vi "Test init from Config file.vi"() -> ()   [LabVIEW 2009, in "POLARIS BME DG.lvlib"]
uses:
  POLARIS BME DG.lvlib
  LV-BME Interface/ChnlSettings.ctl
  DG Classes/BME_DG_System/BME_DG_System.lvclass
  DG Classes/BME_DG_Base/BME_DG_Base.lvclass
  DG Classes/BME_DG_Chnl/BME_DG_Chnl.lvclass
panel:
  out "Created new":bool
  in  "pathCalFiles":path
  in  "pathParameterFile":path
  out "stop error":errorcluster
  out "Problem Chnls out":string[](array[string])
  out "DelayFormulas":string[](array[string])=[" 10000.0095", "Delay Offset +0.819", "Pulspicker On + 0.013"]
  in  "Reset Error":bool
  out "error out":errorcluster
  in  "Update Delay formula":bool=TRUE
  in  "DelayFormula":string=" 10000.0095"
  in  "Aknowledge interrupts":bool=TRUE
  in  "stop 3":bool=TRUE
  in  "SetDelay":bool=TRUE
  in  "UpdateChnl":bool=TRUE
  in  "ChnlParameter":T2 {"ChnParam2write"."Delay (µs)" min=0.0 max=100000000.0 format="%.5f"}
  out "CountsRemains":i32=2147483647
  out "TriggerCounters":i32[](array[numeric])=[281, 0, 0, 0, -533591008, 0, 0, 0, 0]
  out "Interrupts":u32[](array[numeric])=[11153, 10240, 10240, 10240, 11008, 11008, 10240, 10240, 10240] format="%b"
  out "RemainingTriggers":T3(array[cluster])=[[{"Time Stamp"=timestamp(3421911180.6875 s since 1904-01-01), "Numeric"=1}, {"Time Stamp"=timestamp(3421911180.6875 s since 1904-01-01), "Numeric"=1}, {"Time Stamp"=timestamp(3421911180.6875 s since 1904-01-01), "Numeric"=1}, {"Time Stamp"=timestamp(3421911180.6875 s since 1904-01-01), "Numeric"=1}, {"Time Stamp"=timestamp(3421911180.6875 s since 1904-01-01), "Numeric"=9}, {"Time Stamp"=timestamp(3421911180.6875 s since 1904-01-01), "Numeric"=1}, {"Time Stamp"=timestamp(3421911180.6875 s since 1904-01-01), "Numeric"=1}, {"Time Stamp"=timestamp(3421911180.6875 s since 1904-01-01), "Numeric"=1}, {"Time Stamp"=timestamp(3421911180.6875 s since 1904-01-01), "Numeric"=1}], [{"Time Stamp"=timestamp(3421911180.6875 s since 1904-01-01), "Numeric"=10}, {"Time Stamp"=timestamp(3421911180.6875 s since 1904-01-01), "Numeric"=1}, {"Time Stamp"=timestamp(3421911180.6875 s since 1904-01-01), "Numeric"=1}, {"Time Stamp"=timestamp(3421911180.6875 s since 1904-01-01), "Numeric"=1}, {"Time Stamp"=timestamp(3421911180.6875 s since 1904-01-01), "Numeric"=9}, {"Time Stamp"=timestamp(3421911180.6875 s since 1904-01-01), "Numeric"=1}, {"Time Stamp"=timestamp(3421911180.6875 s since 1904-01-01), "Numeric"=1}, {"Time Stamp"=timestamp(3421911180.6875 s since 1904-01-01), "Numeric"=1}, {"Time Stamp"=timestamp(3421911180.6875 s since 1904-01-01), "Numeric"=1}], [{"Time Stamp"=timestamp(3421911180.6875 s since 1904-01-01), "Numeric"=10}, {"Time Stamp"=timestamp(3421911180.6875 s since 1904-01-01), "Numeric"=1}, {"Time Stamp"=timestamp(3421911180.6875 s since 1904-01-01), "Numeric"=1}, {"Time Stamp"=timestamp(3421911180.6875 s since 1904-01-01), "Numeric"=1}, {"Time Stamp"=timestamp(3421911180.6875 s since 1904-01-01), "Numeric"=609}, {"Time Stamp"=timestamp(3421911180.6875 s since 1904-01-01), "Numeric"=1}, {"Time Stamp"=timestamp(3421911180.6875 s since 1904-01-01), "Numeric"=1}, {"Time Stamp"=timestamp(3421911180.6875 s since 1904-01-01), "Numeric"=1}, {"Time Stamp"=timestamp(3421911180.6875 s since 1904-01-01), "Numeric"=1}]] {"Time Stamp" format="%<%I:%M:%S%3u %p>T"}
  in  "stop 2":bool=TRUE
  in  "ReadStatus":bool=TRUE
  in  "Activate":bool=TRUE
  in  "ResetModuloCounters":bool=TRUE
  in  "TriggerModulo":u32=4
  out "Modulo Settings":u32[](array[numeric])=[1, 10, 10]
  out "Chnls":T1[](array[typedef])=[{" Delay (µs)"=10000.0095, "On?"=TRUE, "PositiveVoltage?"=TRUE, "50OhmTerminated? "=TRUE, "25OhmOutput?"=FALSE}, {" Delay (µs)"=10000.829, "On?"=TRUE, "PositiveVoltage?"=TRUE, "50OhmTerminated? "=TRUE, "25OhmOutput?"=FALSE}, {" Delay (µs)"=10000.843, "On?"=TRUE, "PositiveVoltage?"=TRUE, "50OhmTerminated? "=TRUE, "25OhmOutput?"=FALSE}] {"Delay (µs)" min=0.0 max=100000000.0 format="%.5f"}
  in  "Selected Chnl":u16(ring) items=["MA", "MB", "MC", "MD", "ME", "MF"]
  in  "Selected Card":u16(ring) items=["Master", "Slave"]
  in  "STOP":bool
  in  "ChnParam2write":T1={" Delay (µs)"=0.0, "On?"=TRUE, "PositiveVoltage?"=TRUE, "50OhmTerminated? "=TRUE, "25OhmOutput?"=FALSE} {"Delay (µs)" min=0.0 max=100000000.0 format="%.5f"}
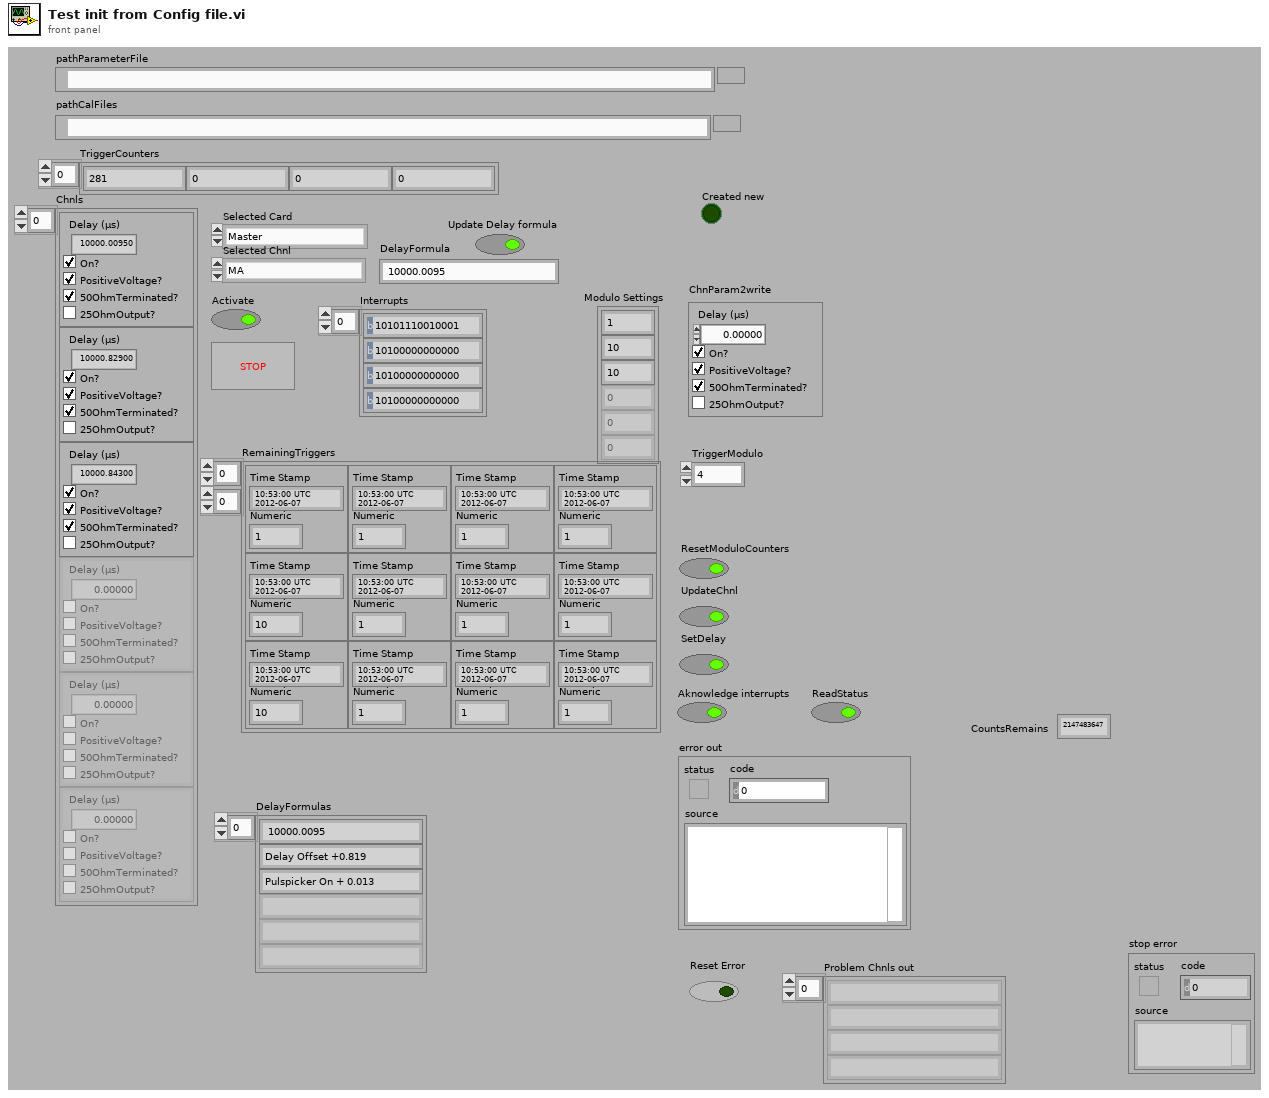
[diagram p1: front panel]
types:
  T1 = typedef "POLARIS BME DG.lvlib/ChnlSettings.ctl" = cluster{" Delay (µs)":dbl, "On?":bool, "PositiveVoltage?":bool, "50OhmTerminated? ":bool, "25OhmOutput?":bool}
  T2 = cluster{"ChnlName":string, "ChnParam2write":T1, "TriggerModulo":u32}
  T3 = cluster{"Time Stamp":timestamp, "Numeric":i32}[][]
  T4 = typedef "POLARIS BME DG.lvlib/BME_DG_MasterOrSlave.ctl" = enum16{"Unknown", "Master", "Slave"}
  T5 = enum8{"Enabled", "Disabled", "Disabled and Grayed Out"}
  T6 = typedef "POLARIS BME DG.lvlib/BME_DG_TriggerSettings.ctl" = cluster{"Clock Source":T7, " clock devide by":u32, "TriggerEnabled?":bool, "Trigger devide by":i32, "InputTerminated?":bool, "Inhibit(µs)":dbl, "TriggerLevel":dbl, "PresetValue":i32, "InternalTrigger?":bool, "InternalArm?":bool, "SWTrigger?":bool, "RisingEdge?":bool, "StopOnPreset?":bool, "ResetWhenDone?":bool, "Gate Divider":i32, "PositiveGate?":bool}
  T7 = typedef "POLARIS BME DG.lvlib/ClockSource.ctl" = i32
  T8 = cluster{"ChnlName":string, "ChnParam2write":T1, "TriggerModulo":u32}[]
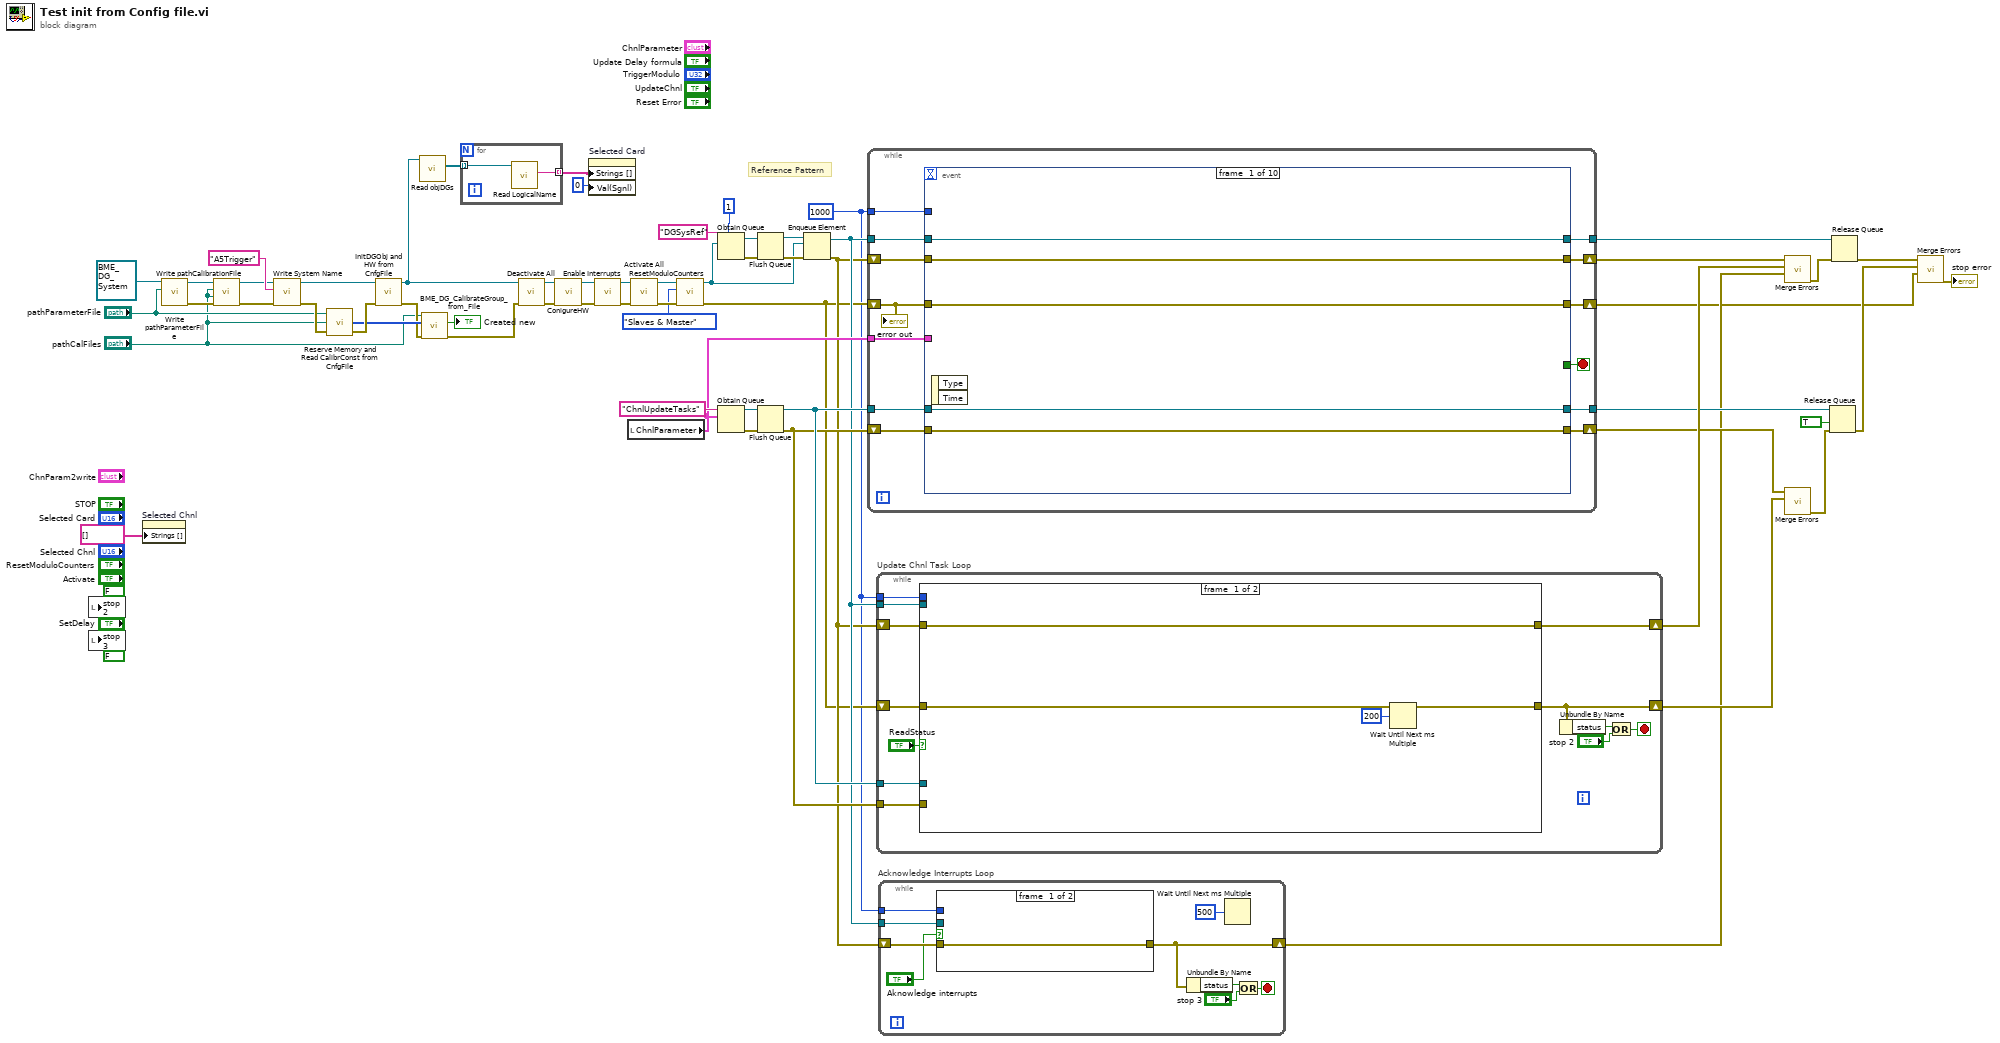
[diagram p0: block diagram]
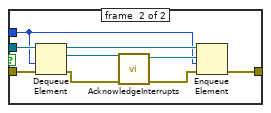
[diagram p2: hidden frame]
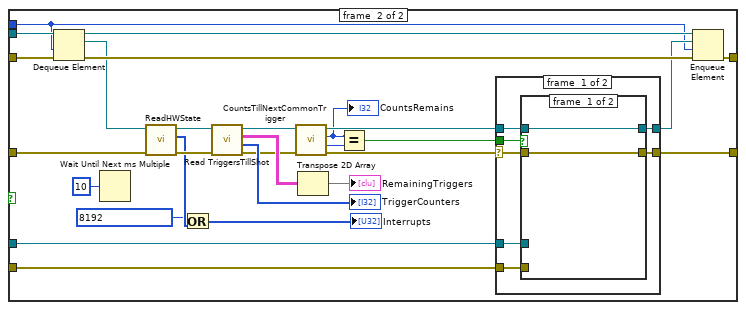
[diagram p3: hidden frame]
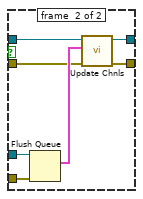
[diagram p4: hidden frame]
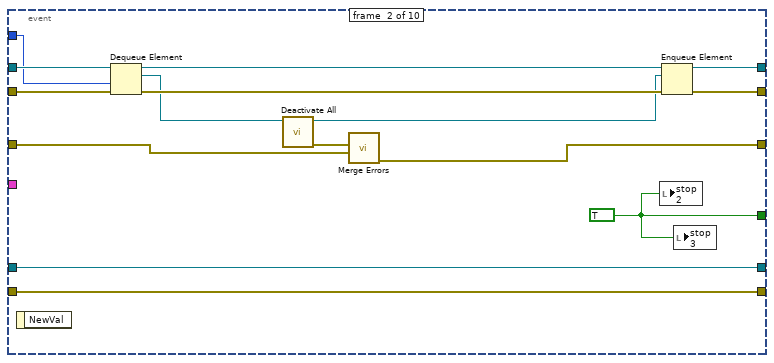
[diagram p6: hidden frame]
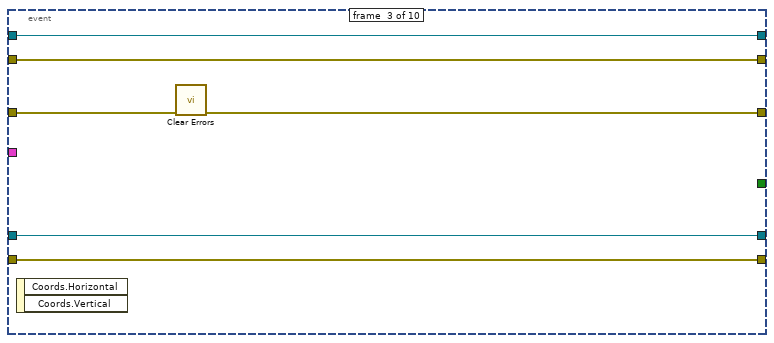
[diagram p7: hidden frame]
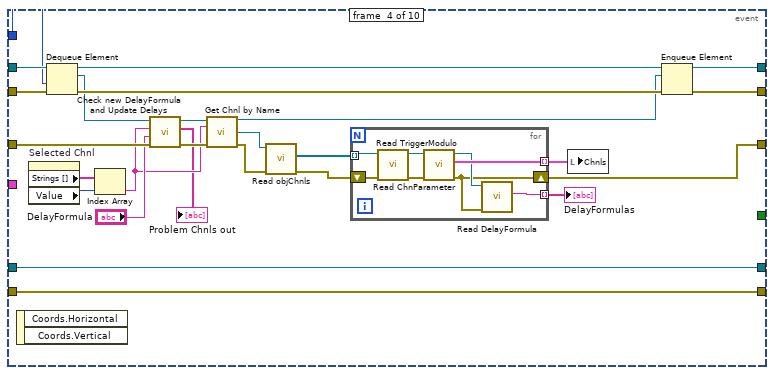
[diagram p8: hidden frame]
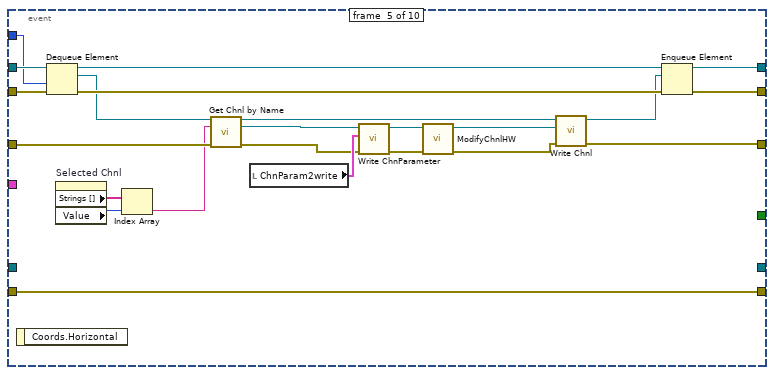
[diagram p9: hidden frame]
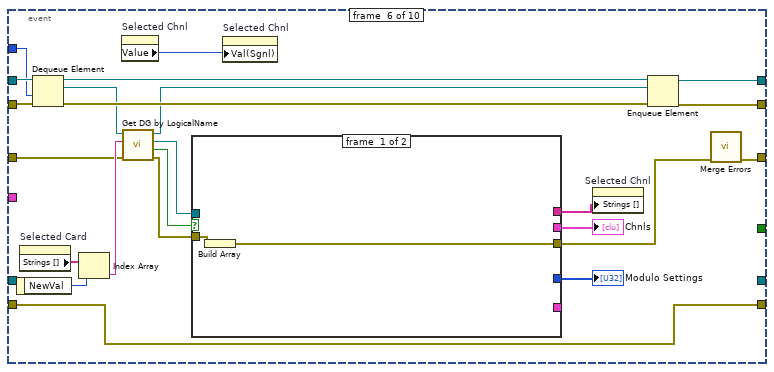
[diagram p10: hidden frame]
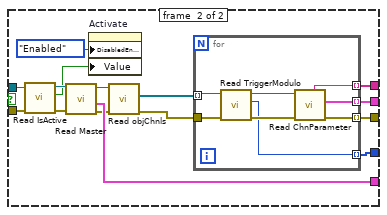
[diagram p11: hidden frame]
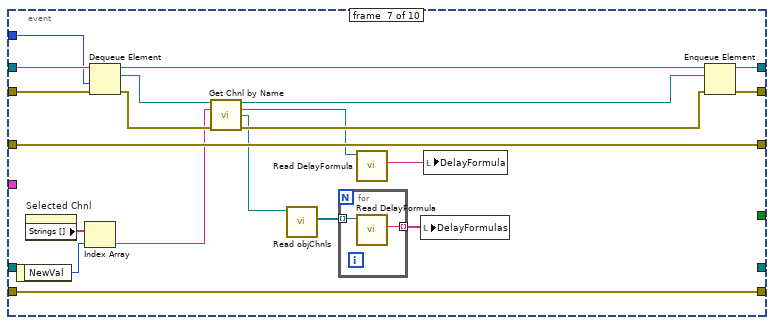
[diagram p12: hidden frame]
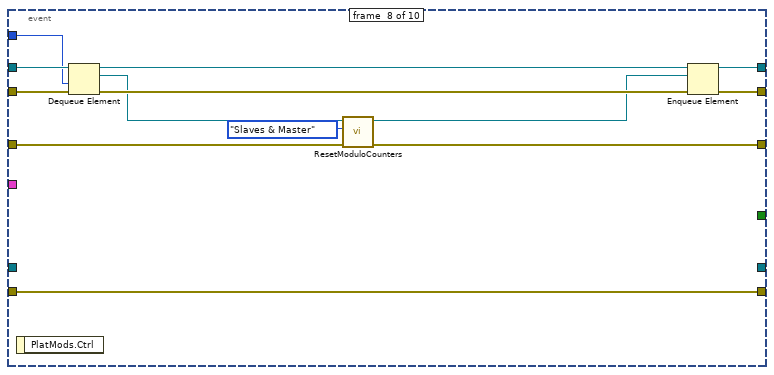
[diagram p13: hidden frame]
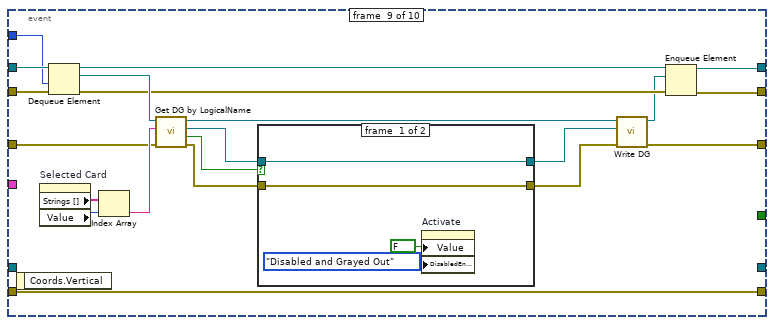
[diagram p14: hidden frame]
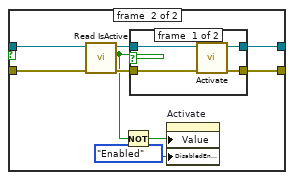
[diagram p15: hidden frame]
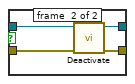
[diagram p16: hidden frame]
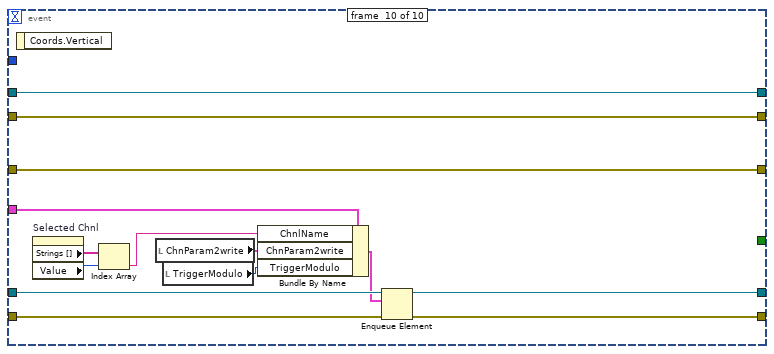
[diagram p17: hidden frame]
diagram:
  w17 = 1000 ("timeout in ms (-1)")
  # "Reference Pattern"
  n1 = local write "stop 2"(FALSE ("stop 2")) -> ()
  n2 = local write "stop 3"(FALSE ("stop 3")) -> ()
  n3 = property on="Selected Chnl" class="Ring (strict)"("Strings []"=string[] []) -> ()  [unwired: 2 in, 2 out]
  n4 = call-dynamic "Write pathParameterFile.vi"("pathParameterFile"="pathParameterFile", "BME_DG_System in"=refnum<class "BME_DG_System.lvclass"> refnum ("BME_DG_System.lvclass")) -> ("error out"=w13:errorcluster, "BME_DG_System out"=w15:refnum<class "BME_DG_System.lvclass">)  [unwired: 8 in]
  n5 = call-dynamic "Write pathCalibrationFile.vi"("error in (no error)"=w13, "pathModulesCal"="pathCalFiles", "pathBMEG0xCal"="pathCalFiles", "BME_DG_System in"=w15) -> ("error out"=w12:errorcluster, "BME_DG_System out"=w14:refnum<class "BME_DG_System.lvclass">)  [unwired: 6 in]
  n6 = call "Write System Name.vi"("error in (no error)"=w12, "log Name"="A5Trigger", "BME_DG_System in"=w14) -> ("error out"=w11:errorcluster, "BME_DG_System out"=w18:refnum<class "BME_DG_System.lvclass">)  [unwired: 7 in]
  n7 = call "Reserve Memory and Read CalibrConst from CnfgFile.vi"("error out 2"=w11, "pathCalibrConsts"="pathCalFiles", "pathConfigFile"="pathParameterFile") -> ("error out"=w10:errorcluster, "Master or Slave?"=w7:T4[])  [unwired: 1 in]
  n8 = call "InitDGObj and HW from CnfgFile.vi"("error in"=w10, "BME_DG_System in"=w18) -> ("error IO"=w6:errorcluster, "BME_DG_System Out"=w3:refnum<class "BME_DG_System.lvclass">)  [unwired: 4 in]
  n9 = call "Read objDGs.vi"("BME_DG_System in"=w3) -> ("objDGs"=w2:refnum<class "BME_DG_Base.lvclass">[])  [unwired: 8 in, 2 out]
  n10 = call "BME_DG_CalibrateGroup_from_File.vi"("error in (no error)"=w6, "p_MasterOrSlave"=w7, "Path"="pathCalFiles") -> ("error out"=w4:errorcluster, "Created new"=→"Created new":bool)  [unwired: 7 in]
  n11 = for {
    tunnel: w2 -> [w64] mode=indexing
    tunnel: [w63] -> w1 mode=indexing
    n12 = call "Read LogicalName.vi"("BME_DG_Base in"=w64) -> ("LogicalName"=w63:string)  [unwired: 8 in, 2 out]
  }
  n13 = call "Deactivate All.vi"("error in (no error)"=w4, "BME_DG_System in"=w3) -> ("error out"=w37:errorcluster, "BME_DG_System out"=w38:refnum<class "BME_DG_System.lvclass">)  [unwired: 8 in]
  n14 = call "ConigureHW.vi"("error in (no error)"=w37, "BME_DG_System in"=w38) -> ("error out"=w35:errorcluster, "BME_DG_System out"=w36:refnum<class "BME_DG_System.lvclass">)  [unwired: 8 in]
  n15 = property on="Selected Card" class="Ring (strict)"("Strings []"=w1, "Val(Sgnl)"=u16 0 ("Value (Signaling)")) -> ()  [unwired: 2 in, 2 out]
  n16 = call "Enable Interrupts.vi"("error in (no error)"=w35, "BME_DG_System in"=w36) -> ("error out"=w29:errorcluster, "BME_DG_System out"=w30:refnum<class "BME_DG_System.lvclass">)  [unwired: 8 in]
  n17 = local read "ChnlParameter"() -> (w46:T2)
  n18 = call "Activate All.vi"("error in (no error)"=w29, "BME_DG_System in"=w30) -> ("error out"=w26:errorcluster, "BME_DG_System out"=w28:refnum<class "BME_DG_System.lvclass">)  [unwired: 8 in]
  n19 = call "ResetModuloCounters.vi"("error in (no error)"=w26, "Enum"=enum16{"Slaves only", "Slaves & Master"}."Slaves & Master", "BME_DG_System in"=w28) -> ("error out"=w25:errorcluster, "BME_DG_System out"=w27:refnum<class "BME_DG_System.lvclass">)  [unwired: 7 in]
  n20 = Obtain Queue(max queue size (-1, unlimited)=1, name (unnamed)="DGSysRef", element data type=w27) -> (queue out=w54:refnum<queue>, error out=w52:errorcluster)  [unwired: 2 in, 1 out]
  n21 = Obtain Queue(name (unnamed)="ChnlUpdateTasks", element data type=w46) -> (queue out=w47:refnum<queue>, error out=w48:errorcluster)  [unwired: 3 in, 1 out]
  n22 = Flush Queue(queue=w54, error in (no error)=w52) -> (queue out=w53:refnum<queue>, error out=w51:errorcluster)  [unwired: 1 out]
  n23 = Flush Queue(queue=w47, error in (no error)=w48) -> (queue out=w43:refnum<queue>, error out=w42:errorcluster)  [unwired: 1 out]
  n24 = Enqueue Element(queue=w53, element=w27, error in (no error)=w51) -> (queue out=w34:refnum<queue>, error out=w33:errorcluster)  [unwired: 1 in, 1 out]
  n25 = while {
    shift-right: [w73] -> w16
    shift-left: w25 -> [w75]
    shift-right: [w71] -> w57
    shift-left: w33 -> [w72]
    tunnel: w34 -> [w76]
    tunnel: [w74] -> w59
    tunnel: w43 -> [w70]
    tunnel: w46 -> [w69]
    tunnel: [w67] -> w45
    shift-right: [w66] -> w41
    shift-left: w42 -> [w68]
    tunnel: w17 -> [w65]
    stop <- w77 stop-if-true
    n26 = event shown="[5] \"Selected Card\": Value Change" {
      selector: _ -> [_ _ _ _ _ _ _ _ _ _]
      dyn-events: _ -> [_ _ _ _ _ _ _ _ _ _]
      timeout: _ -> [_ _ _ _ _ _ _ _ _ _]
      tunnel: [_ w86 _ _ _ _ _ _ _ _] -> w77
      tunnel: w76 -> [w82 w95 w102 w128 w159 w172 w223 w243 w253 w299]
      tunnel: w75 -> [w81 w84 w103 w120 w150 w180 w228 w233 w261 w298]
      tunnel: [w82 w91 w102 w124 w155 w170 w221 w238 w247 w299] -> w74
      tunnel: [w81 w85 w98 w108 w139 w165 w228 w234 w254 w298] -> w73
      tunnel: w72 -> [w80 w94 w101 w127 w158 w171 w222 w241 w252 w295]
      tunnel: [w80 w92 w101 w125 w156 w169 w220 w239 w246 w295] -> w71
      tunnel: w70 -> [w79 w88 w100 w123 _ _ _ _ _ w290]
      tunnel: w69 -> [_ _ _ _ _ _ _ _ _ w294]
      tunnel: w68 -> [w78 w87 w99 w122 w154 w163 w227 w237 w245 w288]
      tunnel: [w79 w88 w100 w123 _ _ _ _ _ w287] -> w67
      tunnel: [w78 w87 w99 w122 w154 w163 w227 w237 w245 w286] -> w66
      tunnel: w65 -> [_ w83 _ w104 w138 w161 w209 w231 w244 _]
      event #0 {
        n27 = event-data() -> ()  [unwired: 1 in, 2 out]
      }
      event #1 {
        w86 = TRUE
        n28 = event-data() -> ()  [unwired: 1 in, 1 out]
        n29 = Dequeue Element(queue=w95, timeout in ms (-1)=w83, error in (no error)=w94) -> (queue out=w96:refnum<queue>, element=w89:refnum<class "BME_DG_System.lvclass">, error out=w93:errorcluster)  [unwired: 1 out]
        n30 = call "Deactivate All.vi"("BME_DG_System in"=w89) -> ("error out"=w97:errorcluster, "BME_DG_System out"=w90:refnum<class "BME_DG_System.lvclass">)  [unwired: 9 in]
        n31 = call <vilib>:"Merge Errors.vi"("error in 3 (no error)"=w84, "error in 2 (no error)"=w97) -> ("error out"=w85:errorcluster)  [unwired: 5 in]
        n32 = local write "stop 2"(w86) -> ()
        n33 = Enqueue Element(queue=w96, element=w90, error in (no error)=w93) -> (queue out=w91:refnum<queue>, error out=w92:errorcluster)  [unwired: 1 in, 1 out]
        n34 = local write "stop 3"(w86) -> ()
      }
      event #2 {
        n35 = event-data() -> ()  [unwired: 1 in, 2 out]
        n36 = call <vilib>:"Clear Errors.vi"("error in (no error)"=w103) -> ("error out"=w98:errorcluster)  [unwired: 6 in]
      }
      event #3 {
        n37 = event-data() -> ()  [unwired: 1 in, 2 out]
        n38 = property on="Selected Chnl" class="Ring (strict)"() -> ("Strings []"=w118:string[], "Value"=w119:u16)  [unwired: 2 in, 2 out]
        n39 = Dequeue Element(queue=w128, timeout in ms (-1)=w104, error in (no error)=w127) -> (queue out=w129:refnum<queue>, element=w121:refnum<class "BME_DG_System.lvclass">, error out=w126:errorcluster)  [unwired: 1 out]
        n40 = Index Array(array=w118, index=w119) -> (element=w107:string)
        n41 = call "Check new DelayFormula and Update Delays.vi"("error in (no error)"=w120, "Delay Formula"="DelayFormula", "ChnlName"=w107, "BME_DG_System in"=w121) -> ("error out"=w110:errorcluster, "Problem Chnls out"=→"Problem Chnls out":string[], "BME_DG_System out"=w112:refnum<class "BME_DG_System.lvclass">)  [unwired: 5 in]
        n42 = call "Get Chnl by Name.vi"("BME_DG_System in"=w112, "Chnl Name"=w107, "error in (no error)"=w110) -> ("BME_DG_System out"=w111:refnum<class "BME_DG_System.lvclass">, "Owner DG"=w113:refnum<class "BME_DG_Base.lvclass">, "error out"=w109:errorcluster)  [unwired: 7 in, 3 out]
        n43 = call-dynamic "Read objChnls.vi"("error in (no error)"=w109, "BME_DG_Base in"=w113) -> ("error out"=w114:errorcluster, "objChnls"=w116:refnum<class "BME_DG_Chnl.lvclass">[])  [unwired: 6 in, 2 out]
        n44 = for {
          tunnel: w116 -> [w136] mode=indexing
          tunnel: [w137] -> w115 mode=indexing
          shift-right: [w131] -> w108
          shift-left: w114 -> [w134]
          tunnel: [w130] -> w106 mode=indexing
          n45 = call-dynamic "Read TriggerModulo.vi"("error in (no error)"=w134, "BME_DG_Chnl in"=w136) -> ("error out"=w133:errorcluster, "BME_DG_Chnl out"=w135:refnum<class "BME_DG_Chnl.lvclass">)  [unwired: 7 in, 1 out]
          n46 = call-dynamic "Read ChnParameter.vi"("error in (no error)"=w133, "BME_DG_Chnl in"=w135) -> ("error out"=w131:errorcluster, "ChnParemater"=w137:T1, "BME_DG_Chnl out"=w132:refnum<class "BME_DG_Chnl.lvclass">)  [unwired: 4 in, 3 out]
          n47 = call-dynamic "Read DelayFormula.vi"("error in (no error)"=w131, "BME_DG_Chnl in"=w132) -> ("DelayFormula"=w130:string)  [unwired: 7 in, 2 out]
        }
        "DelayFormulas" <- w106
        n48 = local write "Chnls"(w115) -> ()
        n49 = Enqueue Element(queue=w129, element=w111, error in (no error)=w126) -> (queue out=w124:refnum<queue>, error out=w125:errorcluster)  [unwired: 1 in, 1 out]
      }
      event #4 {
        n50 = event-data() -> ()  [unwired: 1 in, 1 out]
        n51 = Dequeue Element(queue=w159, timeout in ms (-1)=w138, error in (no error)=w158) -> (queue out=w160:refnum<queue>, element=w151:refnum<class "BME_DG_System.lvclass">, error out=w157:errorcluster)  [unwired: 1 out]
        n52 = property on="Selected Chnl" class="Ring (strict)"() -> ("Strings []"=w152:string[], "Value"=w153:u16)  [unwired: 2 in, 2 out]
        n53 = Index Array(array=w152, index=w153) -> (element=w149:string)
        n54 = call "Get Chnl by Name.vi"("BME_DG_System in"=w151, "Chnl Name"=w149, "error in (no error)"=w150) -> ("BME_DG_System out"=w145:refnum<class "BME_DG_System.lvclass">, "BME_DG_Chnl"=w148:refnum<class "BME_DG_Chnl.lvclass">, "error out"=w146:errorcluster)  [unwired: 7 in, 3 out]
        n55 = local read "ChnParam2write"() -> (w147:T1)
        n56 = call-dynamic "Write ChnParameter.vi"("error in (no error)"=w146, "ChnParemater"=w147, "BME_DG_Chnl in"=w148) -> ("error out"=w142:errorcluster, "BME_DG_Chnl out"=w143:refnum<class "BME_DG_Chnl.lvclass">)  [unwired: 7 in]
        n57 = call-dynamic "ModifyChnlHW.vi"("error in (no error)"=w142, "BME_DG_Chnl in"=w143) -> ("error out"=w140:errorcluster, "BME_DG_Chnl out"=w141:refnum<class "BME_DG_Chnl.lvclass">)  [unwired: 8 in]
        n58 = call "Write Chnl.vi"("error in (no error)"=w140, "BME_DG_Chnl.lvclass"=w141, "BME_DG_System in"=w145) -> ("error out"=w139:errorcluster, "BME_DG_System out"=w144:refnum<class "BME_DG_System.lvclass">)  [unwired: 7 in]
        n59 = Enqueue Element(queue=w160, element=w144, error in (no error)=w157) -> (queue out=w155:refnum<queue>, error out=w156:errorcluster)  [unwired: 1 in, 1 out]
      }
      event #5 {
        n60 = event-data() -> ("NewVal"=w182:u16)  [unwired: 1 in]
        n61 = property on="Selected Card" class="Ring (strict)"() -> ("Strings []"=w183:string[])  [unwired: 2 in, 2 out]
        n62 = Dequeue Element(queue=w172, timeout in ms (-1)=w161, error in (no error)=w171) -> (queue out=w173:refnum<queue>, element=w168:refnum<class "BME_DG_System.lvclass">, error out=w174:errorcluster)  [unwired: 1 out]
        n63 = Index Array(array=w183, index=w182) -> (element=w181:string)
        n64 = property on="Selected Chnl" class="Ring (strict)"() -> ("Value"=w162:u16)  [unwired: 2 in, 2 out]
        n65 = call "Get DG by LogicalName.vi"("error in (no error)"=w180, "LogicalName"=w181, "BME_DG_System in"=w168) -> ("error out"=w166:errorcluster, "found?"=w179:bool, "BME_DG_Base.lvclass"=w178:refnum<class "BME_DG_Base.lvclass">, "BME_DG_System out"=w167:refnum<class "BME_DG_System.lvclass">)  [unwired: 5 in]
        n66 = case shown="True" w179 {
          tunnel: w178 -> [_ w193]
          tunnel: [_ w200] -> w177
          tunnel: [_ w199] -> w176
          tunnel: [_ w198] -> _
          tunnel: [_ w194] -> w175
          tunnel: w166 -> [w185 w190]
          tunnel: [w184 w188] -> w164
          frame #0 {
            n67 = Build Array(w185) -> (w184:errorcluster[])
          }
          frame #1 {
            n68 = call-dynamic "Read IsActive.vi"("error in (no error)"=w190, "BME_DG_Base in"=w193) -> ("error out"=w191:errorcluster, "Active?"=w186:bool, "BME_DG_Base out"=w192:refnum<class "BME_DG_Base.lvclass">)  [unwired: 7 in]
            n69 = call-dynamic "Read Master.vi"("error in (no error)"=w191, "BME_DG_Base in"=w192) -> ("error out"=w195:errorcluster, "TriggerSettings"=w198:T6, "BME_DG_Base out"=w196:refnum<class "BME_DG_Base.lvclass">)  [unwired: 6 in, 1 out]
            n70 = property on="Activate" class="Bool (strict)"("DisabledEnum"=T5."Enabled" ("Disabled"), "Value"=w186) -> ()  [unwired: 2 in, 2 out]
            n71 = call-dynamic "Read objChnls.vi"("error in (no error)"=w195, "BME_DG_Base in"=w196) -> ("error out"=w189:errorcluster, "objChnls"=w197:refnum<class "BME_DG_Chnl.lvclass">[])  [unwired: 6 in, 2 out]
            n72 = for {
              tunnel: w197 -> [w206] mode=indexing
              tunnel: [w208] -> w200 mode=indexing
              tunnel: [w207] -> w199 mode=indexing
              tunnel: [w201] -> w194 mode=indexing
              tunnel: w189 -> [w204]
              tunnel: [w202] -> w188 mode=indexing
              n73 = call-dynamic "Read TriggerModulo.vi"("error in (no error)"=w204, "BME_DG_Chnl in"=w206) -> ("error out"=w203:errorcluster, "TriggerModulo"=w201:i32, "BME_DG_Chnl out"=w205:refnum<class "BME_DG_Chnl.lvclass">)  [unwired: 7 in]
              n74 = call-dynamic "Read ChnParameter.vi"("error in (no error)"=w203, "BME_DG_Chnl in"=w205) -> ("error out"=w202:errorcluster, "ChnParemater"=w207:T1, "Name"=w208:string)  [unwired: 4 in, 3 out]
            }
          }
        }
        "Chnls" <- w176
        "Modulo Settings" <- w175
        n75 = property on="Selected Chnl" class="Ring (strict)"("Val(Sgnl)"=w162) -> ()  [unwired: 2 in, 2 out]
        n76 = property on="Selected Chnl" class="Ring (strict)"("Strings []"=w177) -> ()  [unwired: 2 in, 2 out]
        n77 = Enqueue Element(queue=w173, element=w167, error in (no error)=w174) -> (queue out=w170:refnum<queue>, error out=w169:errorcluster)  [unwired: 1 in, 1 out]
        n78 = call <vilib>:"Merge Errors.vi"("error array in"=w164) -> ("error out"=w165:errorcluster)  [unwired: 6 in]
      }
      event #6 {
        n79 = event-data() -> ("NewVal"=w225:u16)  [unwired: 1 in]
        n80 = property on="Selected Chnl" class="Ring (strict)"() -> ("Strings []"=w226:string[])  [unwired: 2 in, 2 out]
        n81 = Index Array(array=w226, index=w225) -> (element=w215:string)
        n82 = Dequeue Element(queue=w223, timeout in ms (-1)=w209, error in (no error)=w222) -> (queue out=w224:refnum<queue>, element=w216:refnum<class "BME_DG_System.lvclass">, error out=w218:errorcluster)  [unwired: 1 out]
        n83 = call "Get Chnl by Name.vi"("BME_DG_System in"=w216, "Chnl Name"=w215, "error in (no error)"=w218) -> ("BME_DG_System out"=w219:refnum<class "BME_DG_System.lvclass">, "BME_DG_Chnl"=w213:refnum<class "BME_DG_Chnl.lvclass">, "Owner DG"=w212:refnum<class "BME_DG_Base.lvclass">, "error out"=w217:errorcluster)  [unwired: 7 in, 2 out]
        n84 = call-dynamic "Read objChnls.vi"("BME_DG_Base in"=w212) -> ("objChnls"=w211:refnum<class "BME_DG_Chnl.lvclass">[])  [unwired: 7 in, 3 out]
        n85 = for {
          tunnel: w211 -> [w230] mode=indexing
          tunnel: [w229] -> w210 mode=indexing
          n86 = call-dynamic "Read DelayFormula.vi"("BME_DG_Chnl in"=w230) -> ("DelayFormula"=w229:string)  [unwired: 8 in, 2 out]
        }
        n87 = call-dynamic "Read DelayFormula.vi"("BME_DG_Chnl in"=w213) -> ("DelayFormula"=w214:string)  [unwired: 8 in, 2 out]
        n88 = local write "DelayFormulas"(w210) -> ()
        n89 = local write "DelayFormula"(w214) -> ()
        n90 = Enqueue Element(queue=w224, element=w219, error in (no error)=w217) -> (queue out=w221:refnum<queue>, error out=w220:errorcluster)  [unwired: 1 in, 1 out]
      }
      event #7 {
        n91 = event-data() -> ()  [unwired: 1 in, 1 out]
        n92 = Dequeue Element(queue=w243, timeout in ms (-1)=w231, error in (no error)=w241) -> (queue out=w242:refnum<queue>, element=w236:refnum<class "BME_DG_System.lvclass">, error out=w240:errorcluster)  [unwired: 1 out]
        n93 = call "ResetModuloCounters.vi"("error in (no error)"=w233, "Enum"=enum16{"Slaves only", "Slaves & Master"}."Slaves & Master", "BME_DG_System in"=w236) -> ("error out"=w234:errorcluster, "BME_DG_System out"=w235:refnum<class "BME_DG_System.lvclass">)  [unwired: 7 in]
        n94 = Enqueue Element(queue=w242, element=w235, error in (no error)=w240) -> (queue out=w238:refnum<queue>, error out=w239:errorcluster)  [unwired: 1 in, 1 out]
      }
      event #8 {
        n95 = event-data() -> ()  [unwired: 1 in, 1 out]
        n96 = property on="Selected Card" class="Ring (strict)"() -> ("Strings []"=w264:string[], "Value"=w263:u16)  [unwired: 2 in, 2 out]
        n97 = Dequeue Element(queue=w253, timeout in ms (-1)=w244, error in (no error)=w252) -> (queue out=w250:refnum<queue>, element=w251:refnum<class "BME_DG_System.lvclass">, error out=w249:errorcluster)  [unwired: 1 out]
        n98 = Index Array(array=w264, index=w263) -> (element=w262:string)
        n99 = call "Get DG by LogicalName.vi"("error in (no error)"=w261, "LogicalName"=w262, "BME_DG_System in"=w251) -> ("error out"=w259:errorcluster, "found?"=w255:bool, "BME_DG_Base.lvclass"=w260:refnum<class "BME_DG_Base.lvclass">, "BME_DG_System out"=w256:refnum<class "BME_DG_System.lvclass">)  [unwired: 5 in]
        n100 = case shown="True" w255 {
          tunnel: w260 -> [w268 w275]
          tunnel: w259 -> [w267 w273]
          tunnel: [w267 w277] -> w258
          tunnel: [w268 w276] -> w257
          frame #0 {
            n101 = property on="Activate" class="Bool (strict)"("Value"=FALSE ("Activate"), "DisabledEnum"=T5."Disabled and Grayed Out" ("Disabled")) -> ()  [unwired: 2 in, 2 out]
          }
          frame #1 {
            n102 = call-dynamic "Read IsActive.vi"("error in (no error)"=w273, "BME_DG_Base in"=w275) -> ("error out"=w272:errorcluster, "Active?"=w271:bool, "BME_DG_Base out"=w274:refnum<class "BME_DG_Base.lvclass">)  [unwired: 7 in]
            n103 = Not(x=w271) -> (.not. x?=w269:bool)
            n104 = case shown="True" w271 {
              tunnel: [w281 w283] -> w277
              tunnel: [w280 w284] -> w276
              tunnel: w274 -> [w279 w285]
              tunnel: w272 -> [w278 w282]
              frame #0 {
                n105 = call-dynamic "Activate.vi"("error in (no error)"=w278, "BME_DG_Base in"=w279) -> ("error out"=w281:errorcluster, "BME_DG_Base out"=w280:refnum<class "BME_DG_Base.lvclass">)  [unwired: 8 in]
              }
              frame #1 {
                n106 = call-dynamic "Deactivate.vi"("error in (no error)"=w282, "BME_DG_Base in"=w285) -> ("error out"=w283:errorcluster, "BME_DG_Base out"=w284:refnum<class "BME_DG_Base.lvclass">)  [unwired: 8 in]
              }
            }
            n107 = property on="Activate" class="Bool (strict)"("Value"=w269, "DisabledEnum"=T5."Enabled" ("Disabled")) -> ()  [unwired: 2 in, 2 out]
          }
        }
        n108 = call "Write DG.vi"("error in (no error)"=w258, "BME_DG_Base"=w257, "BME_DG_System in"=w256) -> ("error out"=w254:errorcluster, "BME_DG_System out"=w248:refnum<class "BME_DG_System.lvclass">)  [unwired: 7 in]
        n109 = Enqueue Element(queue=w250, element=w248, error in (no error)=w249) -> (queue out=w247:refnum<queue>, error out=w246:errorcluster)  [unwired: 1 in, 1 out]
      }
      event #9 {
        n110 = event-data() -> ()  [unwired: 1 in, 1 out]
        n111 = property on="Selected Chnl" class="Ring (strict)"() -> ("Strings []"=w296:string[], "Value"=w297:u16)  [unwired: 2 in, 2 out]
        n112 = Index Array(array=w296, index=w297) -> (element=w293:string)
        n113 = local read "ChnParam2write"() -> (w292:T1)
        n114 = local read "TriggerModulo"() -> (w291:u32)
        n115 = Bundle By Name(cluster=w294, "ChnlName"=w293, "ChnParam2write"=w292, "TriggerModulo"=w291) -> (w289:T2)
        n116 = Enqueue Element(queue=w290, element=w289, error in (no error)=w288) -> (queue out=w287:refnum<queue>, error out=w286:errorcluster)  [unwired: 1 in, 1 out]
      }
    }
    "error out" <- w75
  }
  n117 = while "Update Chnl Task Loop" {
    tunnel: w34 -> [w308]
    shift-right: [w306] -> w56
    shift-left: w33 -> [w307]
    shift-right: [w303] -> w40
    shift-left: w25 -> [w305]
    tunnel: w43 -> [w302]
    tunnel: w42 -> [w301]
    tunnel: w17 -> [w300]
    stop <- w310 stop-if-true
    n118 = case shown="True" "ReadStatus" {
      tunnel: w308 -> [_ w340]
      tunnel: w307 -> [w313 w339]
      tunnel: [w313 w338] -> w306
      tunnel: w305 -> [w312 w336]
      tunnel: [w312 w322] -> w303
      tunnel: w302 -> [_ w326]
      tunnel: w301 -> [_ w325]
      tunnel: w300 -> [_ w315]
      frame #0 {
        n119 = Wait Until Next ms Multiple(millisecond multiple=u32 200) -> ()  [unwired: 1 out]
      }
      frame #1 {
        n120 = Dequeue Element(queue=w340, timeout in ms (-1)=w315, error in (no error)=w339) -> (queue out=w341:refnum<queue>, element=w337:refnum<class "BME_DG_System.lvclass">, error out=w342:errorcluster)  [unwired: 1 out]
        n121 = Wait Until Next ms Multiple(millisecond multiple=u32 10) -> ()  [unwired: 1 out]
        n122 = call "ReadHWState.vi"("error in (no error)"=w336, "BME_DG_System in"=w337) -> ("error out"=w335:errorcluster, "Interrupts"=w331:u32[], "BME_DG_System out"=w334:refnum<class "BME_DG_System.lvclass">)  [unwired: 7 in]
        n123 = Or(x=u32 8192, y=w331) -> (x .or. y?=→"Interrupts":u32[])
        n124 = call "Read TriggersTillShot.vi"("error in (no error)"=w335, "BME_DG_System in"=w334) -> ("error out"=w327:errorcluster, "TriggerCounters"=→"TriggerCounters":i32[], "RemainingTriggers"=w333:T3, "BME_DG_System out"=w328:refnum<class "BME_DG_System.lvclass">)  [unwired: 6 in]
        n125 = call "CountsTillNextCommonTrigger.vi"("error in (no error)"=w327, "BME_DG_System in"=w328) -> ("error out"=w324:errorcluster, "LeastCommonMult"=w319:i32, "CountsRemains"=w320:i32, "BME_DG_System out"=w323:refnum<class "BME_DG_System.lvclass">)  [unwired: 6 in]
        "CountsRemains" <- w320
        n126 = Transpose 2D Array(2D array=w333) -> (transposed array=→"RemainingTriggers":T3)
        n127 = Equal?(x=w320, y=w319) -> (x = y?=w318:bool)
        n128 = case shown="No Error" w324 {
          selector: w324 -> [w346 w359]
          tunnel: w326 -> [w349 _]
          tunnel: w325 -> [w348 _]
          tunnel: w323 -> [w347 w360]
          tunnel: [w345 w359] -> w322
          tunnel: [w344 w360] -> w321
          tunnel: w318 -> [w343 _]
          frame #0 {
            n129 = case shown="True" w343 {
              tunnel: w349 -> [_ w358]
              tunnel: w348 -> [_ w357]
              tunnel: w347 -> [w351 w356]
              tunnel: w346 -> [w350 w354]
              tunnel: [w350 w353] -> w345
              tunnel: [w351 w352] -> w344
              frame #0 {
              }
              frame #1 {
                n130 = Flush Queue(queue=w358, error in (no error)=w357) -> (remaining elements=w355:T8)  [unwired: 2 out]
                n131 = call "Update Chnls.vi"("error in (no error)"=w354, "ChnlSettings"=w355, "BME_DG_System in"=w356) -> ("error out"=w353:errorcluster, "BME_DG_System out"=w352:refnum<class "BME_DG_System.lvclass">)  [unwired: 7 in]
              }
            }
          }
          frame #1 {
          }
        }
        n132 = Enqueue Element(queue=w341, element=w321, timeout in ms (-1)=w315, error in (no error)=w342) -> (error out=w338:errorcluster)  [unwired: 2 out]
      }
    }
    n133 = Unbundle By Name(w303) -> ("status"=w309:bool)
    n134 = Or(x=w309, y="stop 2") -> (x .or. y?=w310:bool)
  }
  n135 = while "Acknowledge Interrupts Loop" {
    tunnel: w34 -> [w366]
    shift-right: [w364] -> w31
    shift-left: w33 -> [w365]
    tunnel: w17 -> [w361]
    stop <- w368 stop-if-true
    n136 = case shown="True" "Aknowledge interrupts" {
      tunnel: w366 -> [_ w379]
      tunnel: w365 -> [w370 w378]
      tunnel: [w370 w377] -> w364
      tunnel: w361 -> [_ w371]
      frame #0 {
      }
      frame #1 {
        n137 = Dequeue Element(queue=w379, timeout in ms (-1)=w371, error in (no error)=w378) -> (queue out=w376:refnum<queue>, element=w375:refnum<class "BME_DG_System.lvclass">, error out=w374:errorcluster)  [unwired: 1 out]
        n138 = call "AcknowledgeInterrupts.vi"("error in (no error)"=w374, "BME_DG_System in"=w375) -> ("error out"=w372:errorcluster, "BME_DG_System out"=w373:refnum<class "BME_DG_System.lvclass">)  [unwired: 8 in]
        n139 = Enqueue Element(queue=w376, element=w373, timeout in ms (-1)=w371, error in (no error)=w372) -> (error out=w377:errorcluster)  [unwired: 2 out]
      }
    }
    n140 = Unbundle By Name(w364) -> ("status"=w367:bool)
    n141 = Wait Until Next ms Multiple(millisecond multiple=u32 500) -> ()  [unwired: 1 out]
    n142 = Or(x=w367, y="stop 3") -> (x .or. y?=w368:bool)
  }
  n143 = call <vilib>:"Merge Errors.vi"("error in 3 (no error)"=w31, "error in 2 (no error)"=w56, "error in 1 (no error)"=w57) -> ("error out"=w58:errorcluster)  [unwired: 4 in]
  n144 = call <vilib>:"Merge Errors.vi"("error in 2 (no error)"=w40, "error in 1 (no error)"=w41) -> ("error out"=w39:errorcluster)  [unwired: 5 in]
  n145 = Release Queue(queue=w45, force destroy? (F)=TRUE, error in (no error)=w39) -> (error out=w22:errorcluster)  [unwired: 2 out]
  n146 = Release Queue(queue=w59, error in (no error)=w58) -> (error out=w23:errorcluster)  [unwired: 1 in, 2 out]
  n147 = call <vilib>:"Merge Errors.vi"("error in 3 (no error)"=w16, "error in 2 (no error)"=w22, "error in 1 (no error)"=w23) -> ("error out"=→"stop error":errorcluster)  [unwired: 4 in]
